vi "New Value Change Subscription.vi"(10 "Ignore Past Updates? (F)":bool, 11 "ValueChangeSubscription In":refnum<class "ValueChangeSubscription.lvclass">) -> (3 "ValueChangeSubscription Out":refnum<class "ValueChangeSubscription.lvclass">)   [LabVIEW 2017, in "SubscriptionPolicy.lvlib" / "ValueChangeSubscription.lvclass"]
uses:
  <vilib>/gpm_packages/@cs/mva-core/Source/SubscriptionPolicy/ValueChangeSubscription/ValueChangeSubscription.lvclass
  <vilib>/gpm_packages/@cs/mva-core/Source/SubscriptionPolicy/ValueChangeSubscription/ValueChangeSubscription.lvclass/ValueChangeSubscription.ctl
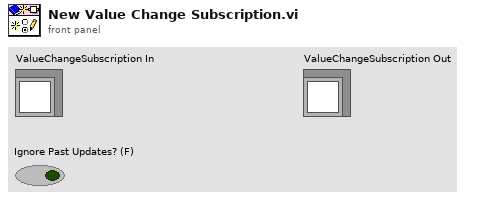
[diagram p1: front panel]
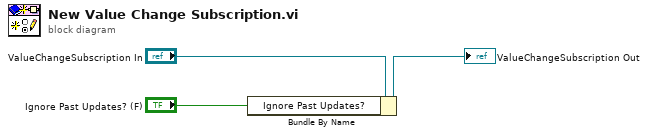
[diagram p0: block diagram]
diagram:
  n1 = Bundle By Name(cluster="ValueChangeSubscription In", "Ignore Past Updates?"="Ignore Past Updates? (F)") -> (→"ValueChangeSubscription Out":refnum<class "ValueChangeSubscription.lvclass">)
